vi "Q_Get Total Distance in KM by Athlete.vi"(8 "error in (no error)":errorcluster, 11 "Data Manager in":refnum<class "Data Manager.lvclass">) -> (0 "error out":errorcluster, 2 "Result Set":string[][](table) caption="Result Set (from first statement with results)", 3 "Data Manager out":refnum<class "Data Manager.lvclass">)   [LabVIEW 2020, in "Data Manager.lvclass"]
uses:
  Data Manager.lvclass
  Data Manager.lvclass/Data Manager.ctl
  <vilib>/drjdpowell/SQLite Library/SQL Connection/Execute SQL.vi
  <vilib>/drjdpowell/SQLite Library/SQLite.lvlib
  <vilib>/drjdpowell/SQLite Library/SQL Connection/Connection.lvclass
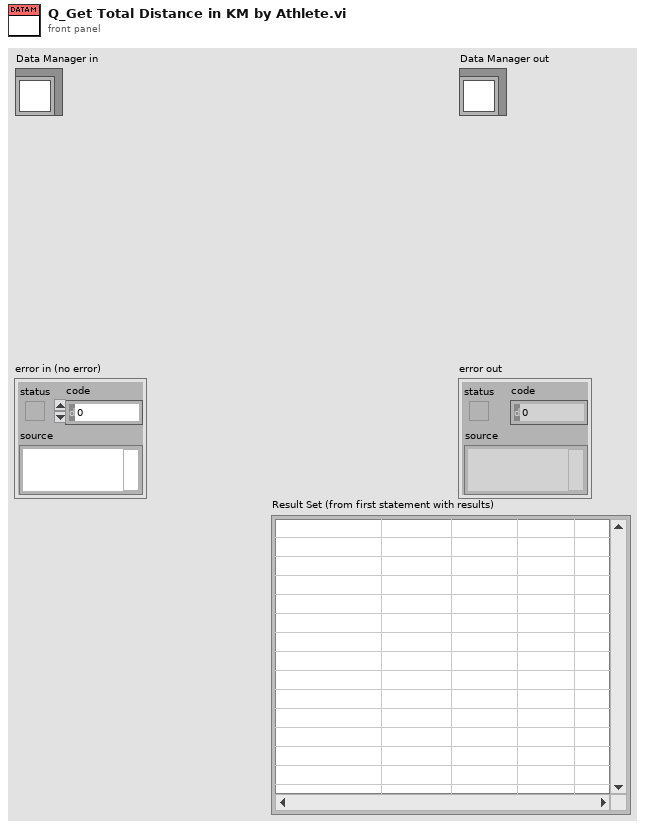
[diagram p1: front panel]
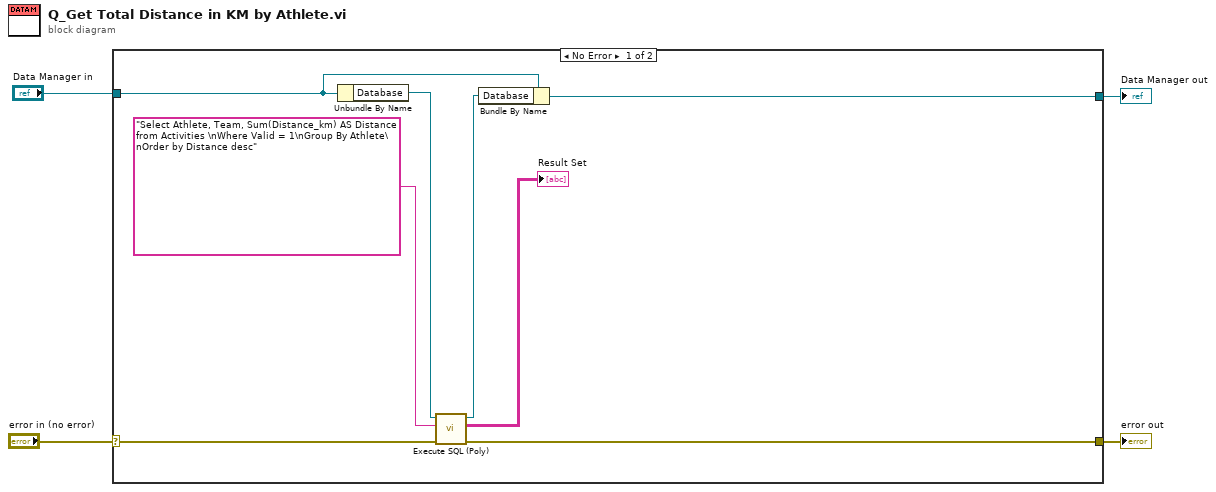
[diagram p0: block diagram]
diagram:
  n1 = case shown="No Error" "error in (no error)" {
    selector: "error in (no error)" -> [w8 w14]
    tunnel: [w7 w14] -> w3
    tunnel: [w10 w13] -> w1
    tunnel: "Data Manager in" -> [w11 w13]
    frame No Error {
      n2 = Unbundle By Name(w11) -> ("Database"=w12:refnum<class "Connection.lvclass">)
      n3 = call-poly <vilib>:"Execute SQL (Poly).vi"("error in (no error)"=w8, "SQL"="Select Athlete, Team, Sum(Distance_km) AS Distance from Activities \nWhere Valid = 1\nGroup By Athlete\nOrder by Distance desc", "SQLite Connection in"=w12) -> ("error out"=w7:errorcluster, "Result Set"=→"Result Set":string[][], "SQLite Connection"=w9:refnum<class "Connection.lvclass">)  [unwired: 5 in, 1 out]
      n4 = Bundle By Name(cluster=w11, "Database"=w9) -> (w10:refnum<class "Data Manager.lvclass">)
    }
    frame Error {
    }
  }
  "error out" <- w3
  "Data Manager out" <- w1
